vi "Pixel_Scan_Engine.vi"(0 "Pixel Scan Parameters In":T2={"Scan Start Pixel"=1, "Scan End Pixel"=1, "Pixel Start Value (-1 to 1)"=-0.5, "Pixel End Value (-1 to 1)"=0.5, "Number of Steps"=0.1}, 1 "DM #":T1(ring), 2 "Action":T3(ring), 11 "Initial Pixel Values (-1 to 1)":dbl[](array[numeric])) -> ()   [LabVIEW 2014]
uses:
  Controls/Pixel Scan Parameters.ctl
  Controls/Standard_Counter_Action.ctl
  Controls/Standard Action.ctl
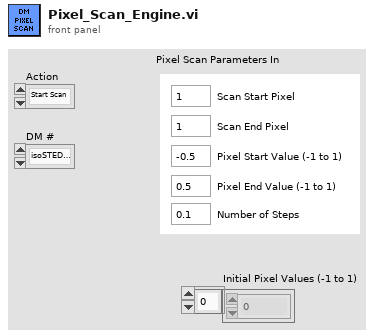
[diagram p1: front panel]
types:
  T1 = enum16{"isoSTED Upper #058", "isoSTED Lower #029"}
  T2 = typedef "Pixel Scan Parameters.ctl" = cluster{"Scan Start Pixel":i32, "Scan End Pixel":i32, "Pixel Start Value (-1 to 1)":dbl, "Pixel End Value (-1 to 1)":dbl, "Number of Steps":dbl}
  T3 = enum16{"Start Scan", "Reset Counter", "Write DM", "Get Image", "Update Count", "Exit"}
  T4 = typedef "Standard_Counter_Action.ctl" = enum16{"Initialize", "Update Count", "Get Count"}
  T5 = typedef "Standard Action.ctl" = enum16{"Read", "Write"}
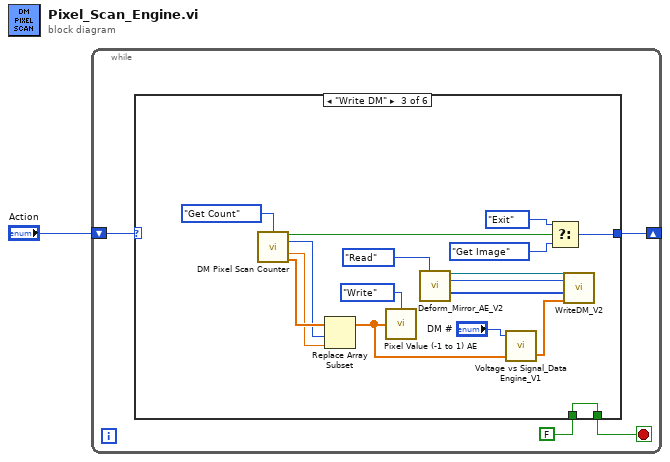
[diagram p0: block diagram]
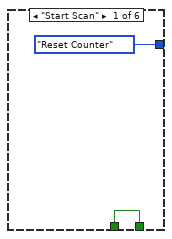
[diagram p2: hidden frame]
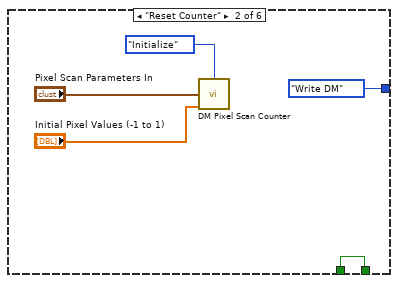
[diagram p3: hidden frame]
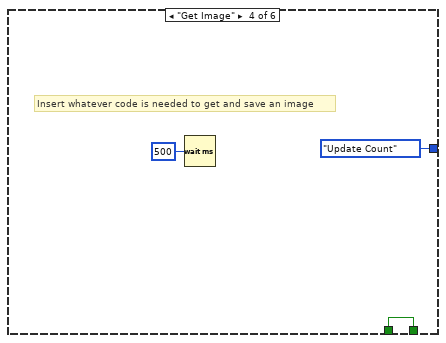
[diagram p4: hidden frame]
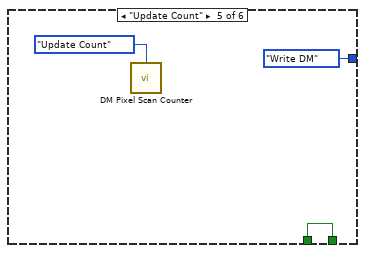
[diagram p5: hidden frame]
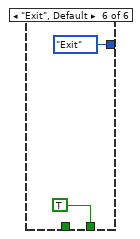
[diagram p6: hidden frame]
diagram:
  n1 = while {
    shift-right: [w2] -> _
    shift-left: "Action" -> [w5]
    stop <- w4 stop-if-true
    n2 = case shown="\"Write DM\"" w5 {
      tunnel: [w7 w9 w19 w32 w34 TRUE] -> w4
      tunnel: FALSE -> [w7 w9 w19 w32 w34 _]
      tunnel: [T3."Reset Counter" ("Action") T3."Write DM" ("Action") w20 T3."Update Count" ("Action") T3."Write DM" ("Action") T3."Exit" ("Action")] -> w2
      frame "Start Scan" {
      }
      frame "Reset Counter" {
        n3 = call "DM Pixel Scan Counter.vi"("Action"=Standard_Counter_Action."Initialize", "Pixel Scan Parameters In"="Pixel Scan Parameters In", "Initial Pixel Values (-1 to 1)"="Initial Pixel Values (-1 to 1)") -> ()  [unwired: 9 in, 4 out]
      }
      frame "Write DM" {
        n4 = call "DM Pixel Scan Counter.vi"("Action"=Standard_Counter_Action."Get Count") -> ("Scan Done"=w21:bool, "DM Pixel"=w26:i32, "Normalized DM Pixel Value"=w25:dbl, "Initial Pixel Values OUT"=w27:dbl[])  [unwired: 11 in]
        n5 = Replace Array Subset(array=w27, new element=w25, index=w26) -> (w15:dbl[])
        n6 = call "Pixel Value (-1 to 1) AE.vi"("Action"=Standard_Action."Write", "Pixel Value (-1 to 1)"=w15) -> ()  [unwired: 13 in, 1 out]
        n7 = call "Deform_Mirror_AE_V2.vi"("Action"=Standard_Action."Read") -> ("Refnum Out"=w22:refnum<k7>, "IDs Out"=w23:i32, "Multi Map Data Out"=w24:i32[])  [unwired: 10 in, 2 out]
        n8 = call "Voltage vs Signal_Data Engine_V1.vi"("Control Signal In (-1~1)"=w15, "DM #"="DM #") -> ("Voltage Out (0~Max. Vol.)"=w14:dbl[])  [unwired: 1 in, 1 out]
        n9 = Select(t=T3."Exit" ("Action"), s=w21, f=T3."Get Image" ("Action")) -> (s? t:f=w20:T3)
        n10 = call "WriteDM_V2.vi"("reference in"=w22, "nDevId"=w23, "MultiDM  Mapping"=w24, "Voltage Array in"=w14) -> ()  [unwired: 2 in, 2 out]
      }
      frame "Get Image" {
        # "Insert whatever code is needed to get and save an image"
        n11 = Wait (ms)(milliseconds to wait=u32 500) -> ()  [unwired: 1 out]
      }
      frame "Update Count" {
        n12 = call "DM Pixel Scan Counter.vi"("Action"=Standard_Counter_Action."Update Count") -> ()  [unwired: 11 in, 4 out]
      }
      frame "Exit", Default {
      }
    }
  }
